vi "Calculated Sector to Speed &Turn Optimizing for Nav.vi"(10 "RAW SICK Data":T1, 11 "Calculated Sector":i16) -> (3 "Motor Commands":T2)   [LabVIEW 2009]
uses:
  Remote Control/Motor Command.ctl
  TypeDefs/Sensor TypeDefs/SICK Array.ctl
panel:
  in  "Turbo Threshold":u16=100
  in  "Max Turn Speed":i16=25
  in  "Minimum Threshold":u16=100
  in  "Axis Turn Speed":i16=10
  out "Error":bool
  in  "Maximum speed":i16=40
  in  "Minimum speed":i16=15
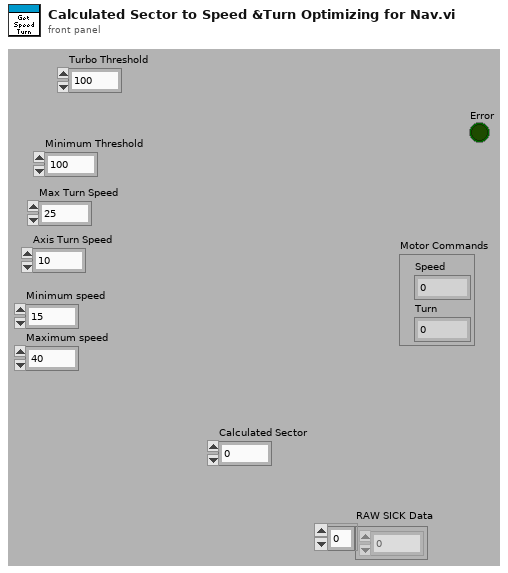
[diagram p1: front panel]
types:
  T1 = typedef "SICK Array.ctl" = u16[]
  T2 = typedef "Motor Command.ctl" = cluster{"Speed":i16, "Turn":i16}
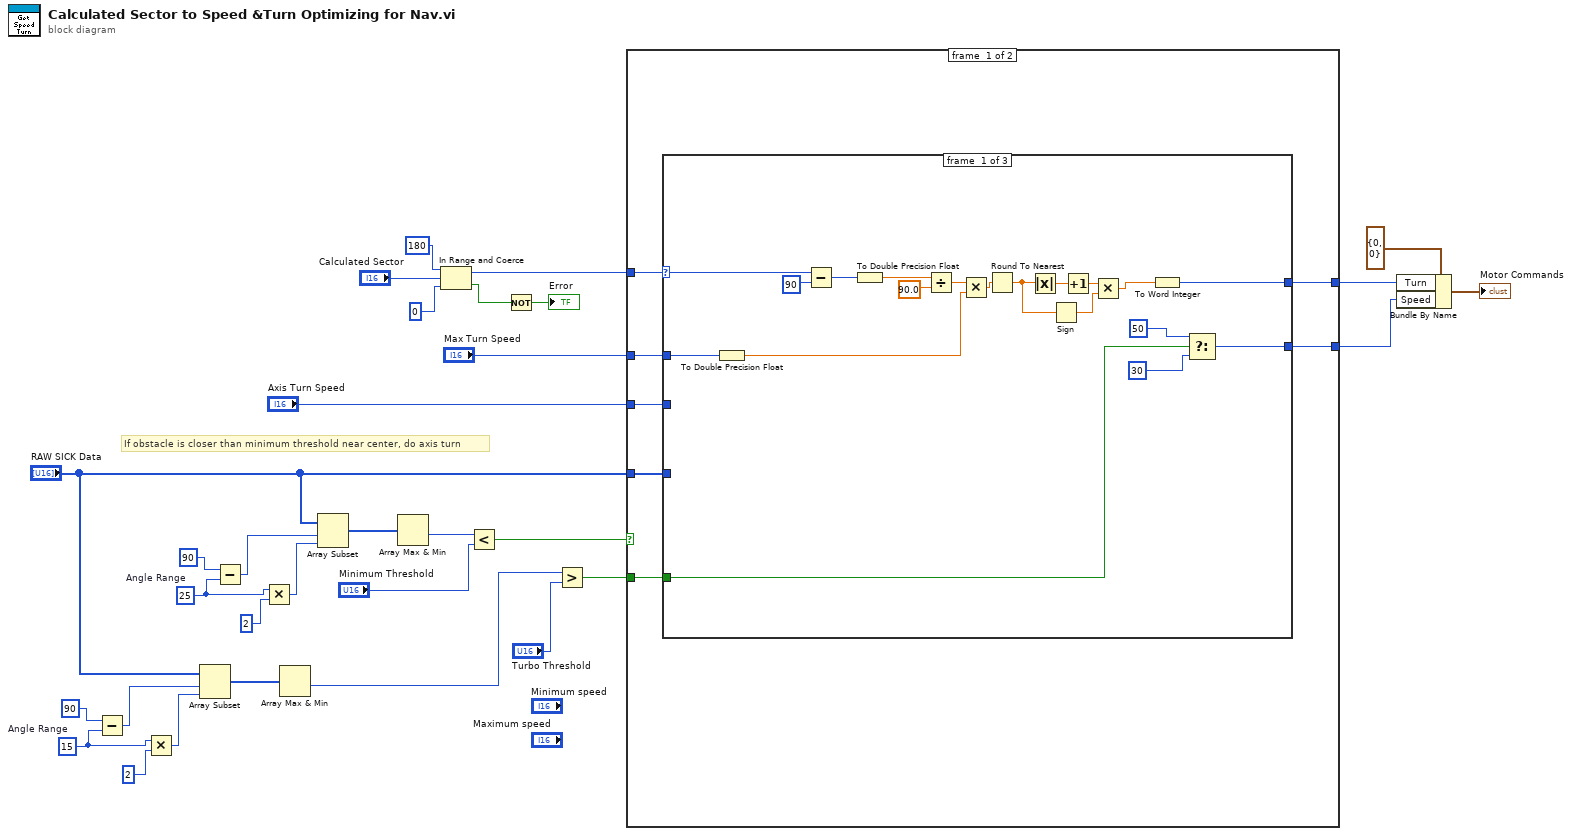
[diagram p0: block diagram]
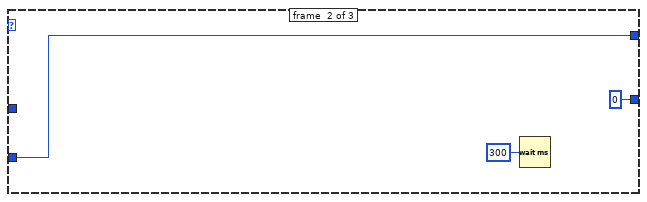
[diagram p2: hidden frame]
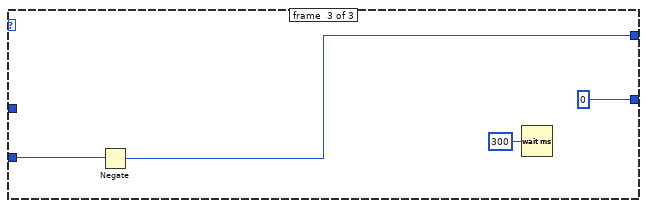
[diagram p3: hidden frame]
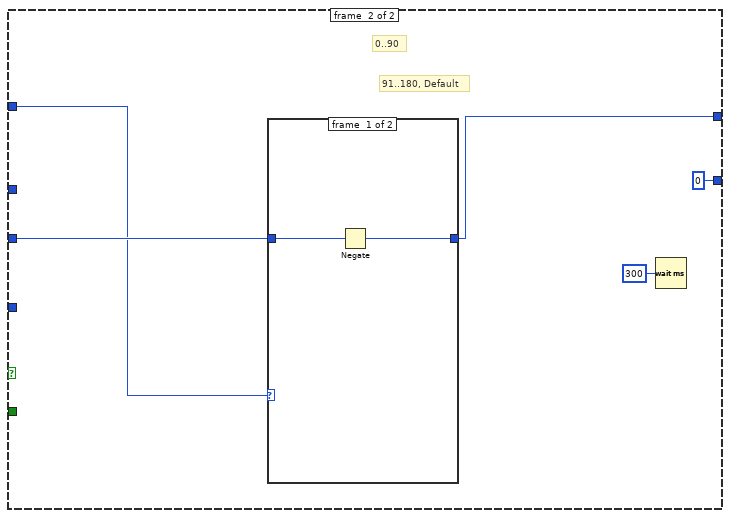
[diagram p4: hidden frame]
diagram:
  w6 = 15  # Angle Range
  w19 = 25  # Angle Range
  # "If obstacle is closer than minimum threshold near center, do axis turn"
  n1 = Subtract(x=90 ("y"), y=w6) -> (x-y=w5:i32)
  n2 = Multiply(x=w6, y=2) -> (x*y=w7:i32)
  n3 = Array Subset(array="RAW SICK Data", index=w5, length=w7) -> (w8:T1)
  n4 = Subtract(x=90 ("y"), y=w19) -> (x-y=w20:i32)
  n5 = Multiply(x=w19, y=2) -> (x*y=w17:i32)
  n6 = Array Max & Min(array=w8) -> (min value=w2:u16)  [unwired: 3 out]
  n7 = Array Subset(array="RAW SICK Data", index=w20, length=w17) -> (w16:T1)
  n8 = Array Max & Min(array=w16) -> (min value=w15:u16)  [unwired: 3 out]
  n9 = In Range and Coerce(upper limit=i16 180, x="Calculated Sector", lower limit=i16 0 ("x")) -> (coerced(x)=w24:i16, In Range?=w23:bool)
  n10 = Less?(x=w15, y="Minimum Threshold") -> (x < y?=w14:bool)
  n11 = Not(x=w23) -> (.not. x?=→"Error":bool)
  n12 = Greater?(x=w2, y="Turbo Threshold") -> (0:w9:bool)
  n13 = case shown="False" w14 {
    tunnel: [w38 i16 0 ("Maximum speed")] -> w30
    tunnel: [w37 w68] -> w28
    tunnel: w24 -> [w36 w66]
    tunnel: "RAW SICK Data" -> [w35 _]
    tunnel: "Axis Turn Speed" -> [w34 w67]
    tunnel: "Max Turn Speed" -> [w33 _]
    tunnel: w9 -> [w32 _]
    frame #0 {
      n14 = case shown="31..149, Default" w36 {
        selector: w36 -> [w51 _ _]
        tunnel: [w40 i16 0 ("Maximum speed") i16 0 ("Maximum speed")] -> w38
        tunnel: w35 -> [_ _ _]
        tunnel: [w52 w59 w62] -> w37
        tunnel: w34 -> [_ w59 w63]
        tunnel: w33 -> [w43 _ _]
        tunnel: w32 -> [w39 _ _]
        frame #0 {
          n15 = To Double Precision Float(number=w43) -> (double precision float=w44:dbl)
          n16 = Subtract(x=w51, y=i16 90) -> (x-y=w53:i16)
          n17 = To Double Precision Float(number=w53) -> (double precision float=w54:dbl)
          n18 = Divide(x=w54, y=90.0) -> (x/y=w55:dbl)
          n19 = Multiply(x=w55, y=w44) -> (x*y=w45:dbl)
          n20 = Round To Nearest(number=w45) -> (nearest integer value=w48:dbl)
          n21 = Absolute Value(x=w48) -> (abs(x)=w50:dbl)
          n22 = Sign(1:w48) -> (0:w47:dbl)
          n23 = Increment(x=w50) -> (x+1=w49:dbl)
          n24 = Multiply(x=w49, y=w47) -> (x*y=w46:dbl)
          n25 = To Word Integer(number=w46) -> (16bit integer=w52:i16)
          n26 = Select(t=i16 50, s=w39, f=i16 30 ("Maximum speed")) -> (s? t:f=w40:i16)
        }
        frame #1 {
          n27 = Wait (ms)(milliseconds to wait=u32 300) -> ()  [unwired: 1 out]
        }
        frame #2 {
          n28 = Negate(x=w63) -> (-x=w62:i16)
          n29 = Wait (ms)(milliseconds to wait=u32 300) -> ()  [unwired: 1 out]
        }
      }
    }
    frame #1 {
      # "0..90"
      # "91..180, Default"
      n30 = case shown="0..90" w66 {
        tunnel: [w70 w72] -> w68
        tunnel: w67 -> [w71 w72]
        frame #0 {
          n31 = Negate(x=w71) -> (-x=w70:i16)
        }
        frame #1 {
        }
      }
      n32 = Wait (ms)(milliseconds to wait=u32 300) -> ()  [unwired: 1 out]
    }
  }
  n33 = Bundle By Name(cluster=T2 {"Speed"=0, "Turn"=0} ("Motor Command"), "Turn"=w28, "Speed"=w30) -> (→"Motor Commands":T2)
